vi "image_encode_base64.vi"(2 "error in (no error)":errorcluster, 3 "imagepaths":path[](array[path])) -> (0 "error out":errorcluster, 1 "image_data":string[](array[string]))   [LabVIEW 2020, in "llm_gemini_chatmodels.lvclass"]
uses:
  llm_gemini_chatmodels.lvclass
  <vilib>/httpClient/LabVIEWHTTPClient.lvlib
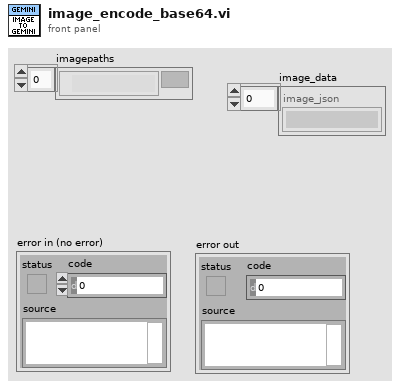
[diagram p1: front panel]
types:
  T1 = cluster{"inline_data":cluster{"mime_type":string, "data":string}}
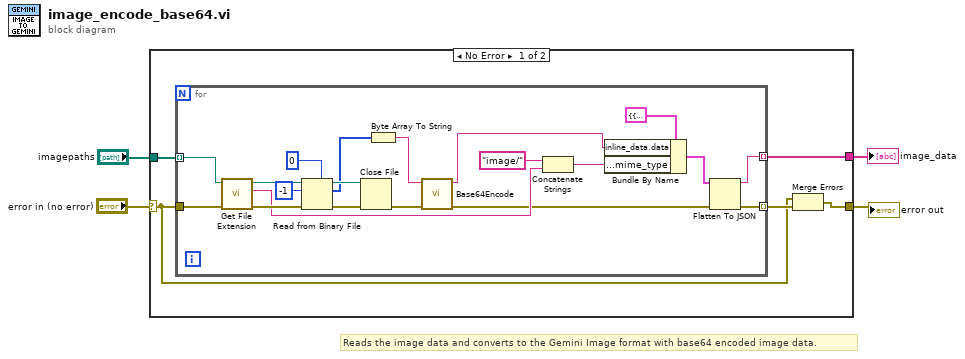
[diagram p0: block diagram]
diagram:
  # "Reads the image data and converts to the Gemini Image format with base64 encoded image data."
  n1 = case shown="No Error" "error in (no error)" {
    selector: "error in (no error)" -> [w5 w30]
    tunnel: [w9 _] -> w4
    tunnel: "imagepaths" -> [w8 _]
    tunnel: [w6 w30] -> w2
    frame No Error {
      n2 = for {
        tunnel: [w16] -> w9 mode=indexing
        tunnel: w8 -> [w20] mode=indexing
        tunnel: [w18] -> w7 mode=indexing
        tunnel: w5 -> [w19]
        n3 = call <vilib>:"Get File Extension.vi"("error in (no error)"=w19, "file"=w20) -> ("error out"=w29:errorcluster, "lowercase file extension"=w22:string, "dup file"=w28:path)  [unwired: 5 in, 2 out]
        n4 = Read from Binary File(5:u8 0 ("unsigned 8bit integer"), 8:w29, 10:-1 ("count (1)"), 11:w28) -> (0:w26:errorcluster, 2:w13:u8[], 3:w27:refnum<file>)  [unwired: 2 in, 1 out]
        n5 = Close File(refnum=w27, error in=w26) -> (error out=w12:errorcluster)  [unwired: 1 out]
        n6 = Byte Array To String(unsigned byte array=w13) -> (string=w14:string)
        n7 = call <vilib>:"Base64Encode.vi"("error in (no error)"=w12, "buffer in"=w14) -> ("error out"=w11:errorcluster, "encoded string"=w10:string)  [unwired: 8 in]
        n8 = Concatenate Strings("image/" ("string"), w22) -> (w21:string)
        n9 = Bundle By Name(cluster=T1 {"inline_data"={"mime_type"="", "data"=""}} ("image_data"), "inline_data.data"=w10, "inline_data.mime_type"=w21) -> (w17:T1)
        n10 = Flatten To JSON(anything=w17, error in (no error)=w11) -> (JSON string=w16:string, 11:w18:errorcluster)  [unwired: 1 in]
      }
      n11 = Merge Errors(w5, w7) -> (w6:errorcluster)
    }
    frame Error {
    }
  }
  "image_data" <- w4
  "error out" <- w2
